vi "IP_Run-Disable.vi"(0 "Base Station":T5, 7 "Element":T4={"Cellular Tect"="", "IP_NETWORK"="BS1", "IP_TYPE"="", "IP_Client Address"="10.45.0.2", "IP_ThgroughPut(Mbps)"=0, "Duration"=0, "Status"=FALSE}, 11 "error in (no error)":errorcluster) -> (4 "Output String":string, 15 "error out":errorcluster)   [LabVIEW 2021]
uses:
  APIs/Controls/Base_Station_Emulator.ctl
  Controls/IP_Cellular Tech Type def.ctl
  Controls/IP_Network_Type def.ctl
  Controls/IP_Type-Tydedef.ctl
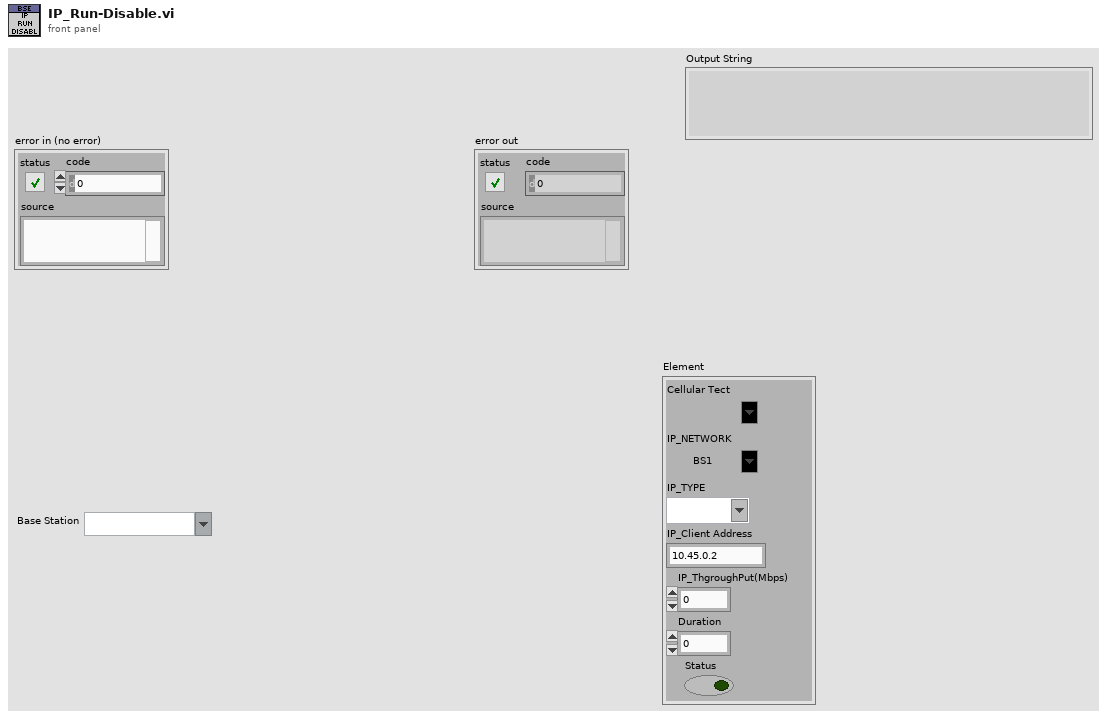
[diagram p1: front panel]
types:
  T1 = typedef "IP_Cellular Tech Type def.ctl" = string
  T2 = typedef "IP_Network_Type def.ctl" = string
  T3 = typedef "IP_Type-Tydedef.ctl" = string
  T4 = cluster{"Cellular Tect":T1, "IP_NETWORK":T2, "IP_TYPE":T3, "IP_Client Address":string, "IP_ThgroughPut(Mbps)":i32, "Duration":i32, "Status":bool}
  T5 = typedef "Base_Station_Emulator.ctl" = string
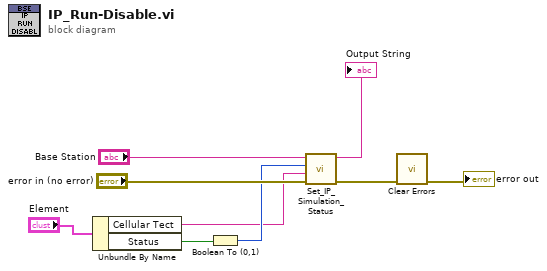
[diagram p0: block diagram]
diagram:
  n1 = Unbundle By Name("Element") -> ("Cellular Tect"=w4:T1, "Status"=w2:bool)
  n2 = Boolean To (0,1)(Boolean=w2) -> (0, 1=w5:i16)
  n3 = call "Set_IP_Simulation_Status.vi"("error in (no error)"="error in (no error)", "Cellular Tech"=w4, "value"=w5, "Base Station"="Base Station") -> ("error out"=w8:errorcluster, "Output String"=→"Output String":string)  [unwired: 6 in]
  n4 = call <vilib>:"Clear Errors.vi"("error in (no error)"=w8) -> ("error out"=→"error out":errorcluster)  [unwired: 5 in, 1 out]
